vi "Configure ARB CDWell Level.vi"(7 "Level-low":dbl min=0.0, 8 "error in":errorcluster, 9 "Level-high":dbl min=0.0, 10 "Step":i32=1 min=1 max=65535, 11 "VISA resource name":refnum<visa-resource-name>) -> (0 "error out":errorcluster, 3 "VISA resource name out":refnum<visa-resource-name>)   [LabVIEW 2015, in "IT-M3900C.lvlib"]
doc: "This command sets the ARB data list.\n<b>Step</b>\n1-65535\n<b>Level-high</b>\n0-MAX\n<b>Level-low</b>\n0-MAX"
uses:
  <instrlib>/IT-M3900C/IT-M3900C.lvlib
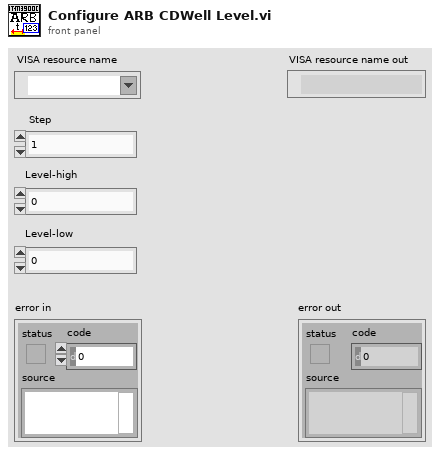
[diagram p1: front panel]
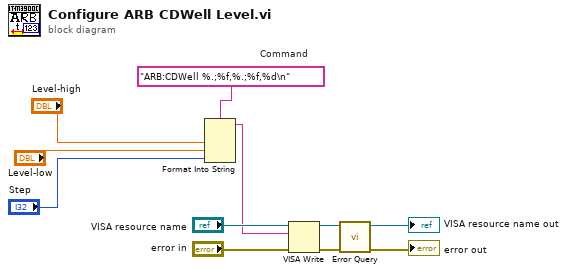
[diagram p0: block diagram]
diagram:
  w5 = "ARB:CDWell %.;%f,%.;%f,%d\n"  # Command
  n1 = Format Into String(format string=w5, "Level-high", "Level-low", "Step") -> (resulting string=w4:string)  [unwired: 2 in, 1 out]
  n2 = VISA Write(VISA resource name="VISA resource name", write buffer=w4, error in (no error)="error in") -> (VISA resource name out=w8:refnum<visa-resource-name>, error out=w9:errorcluster)  [unwired: 1 out]
  n3 = call <instrlib>:"Error Query.vi"("error in"=w9, "VISA resource name"=w8) -> ("error out"=→"error out":errorcluster, "VISA resource name out"=→"VISA resource name out":refnum<visa-resource-name>)  [unwired: 6 in, 2 out]
